vi "emi_Is VI Running.vi"(5 "VI reference":refnum<vi>, 9 "error in (no error)":errorcluster) -> (6 "reference out":refnum<vi>, 8 "Running?":bool, 10 "error out":errorcluster)   [LabVIEW 2010]
doc: "Check if a VI is running or not based on refrence.\n\nUse Vi propery Exec.State. If it is Eiterh Running, or Run Top Level, Vi returns true.\n\nIf VI refrence is not valid. Returns false and an error.\n\nON Error: No Action, returns false."
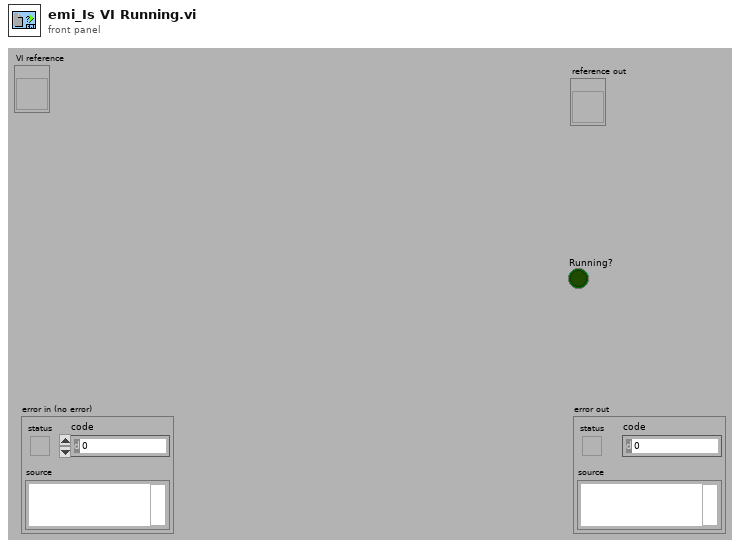
[diagram p1: front panel]
types:
  T1 = enum32{"Bad", "Idle", "Run top level", "Running"}
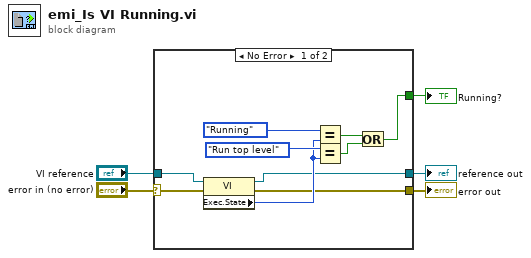
[diagram p0: block diagram]
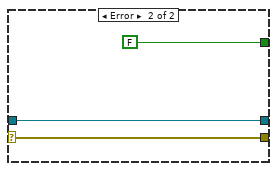
[diagram p2: hidden frame]
diagram:
  n1 = case shown="No Error" "error in (no error)" {
    selector: "error in (no error)" -> [w6 w17]
    tunnel: [w15 FALSE] -> w5
    tunnel: [w9 w18] -> w4
    tunnel: "VI reference" -> [w8 w18]
    tunnel: [w7 w17] -> w2
    frame No Error {
      n2 = property class="VI"(reference=w8, error in=w6) -> (reference out=w9:refnum<vi>, error out=w7:errorcluster, "Exec.State"=w11:T1)
      n3 = Equal?(x=T1."Running" ("Execution:State"), y=w11) -> (x = y?=w13:bool)
      n4 = Equal?(x=T1."Run top level" ("Execution:State"), y=w11) -> (x = y?=w14:bool)
      n5 = Or(x=w13, y=w14) -> (x .or. y?=w15:bool)
    }
    frame Error {
    }
  }
  "error out" <- w2
  "reference out" <- w4
  "Running?" <- w5
